vi "DiscardData.vi"(8 "error in (no err)":errorcluster caption="entrée d'erreur (pas d'erreur)", 11 "Interface In":refnum<class "Interface.lvclass"> caption="DNL_LabVIEW Object in") -> (0 "error out":errorcluster caption="sortie d'erreur", 3 "Interface Out":refnum<class "Interface.lvclass"> caption="DNL_LabVIEW Object out")   [LabVIEW 2019, in "Interface.lvclass"]
uses:
  Interface.lvclass
  Interface.lvclass/Interface.ctl
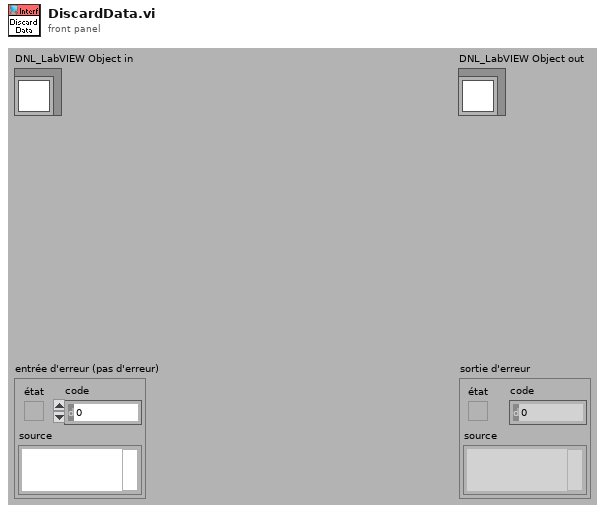
[diagram p1: front panel]
types:
  T1 = typedef "Interface.lvclass/CurveSetup.ctl" = cluster{"CurveName":string, "YParam":string, "XParam":string, "ZParam ":string, "GroupName":string, "LinWdth":u8, "PntCol":u32, "LinCol":u32, "LablFor":u8, "XScale":u32, "YScale":u32, "Interpol":u8, "DisplayName":string, "FillType":i16, "LineStyle":u8, "PntStyle":u8, "BarTyp":u8, "GraphIndex":i32, "Visible":bool, "XScaleName":string, "YScaleName":string, "XYGraph_Ref":refnum<vi>, "Data Only":bool, "DataQ Ref":refnum<queue>, "XParQ Ref":refnum<queue>, "XParamInd":i32, "ScanInd":i32, "File Path":path}
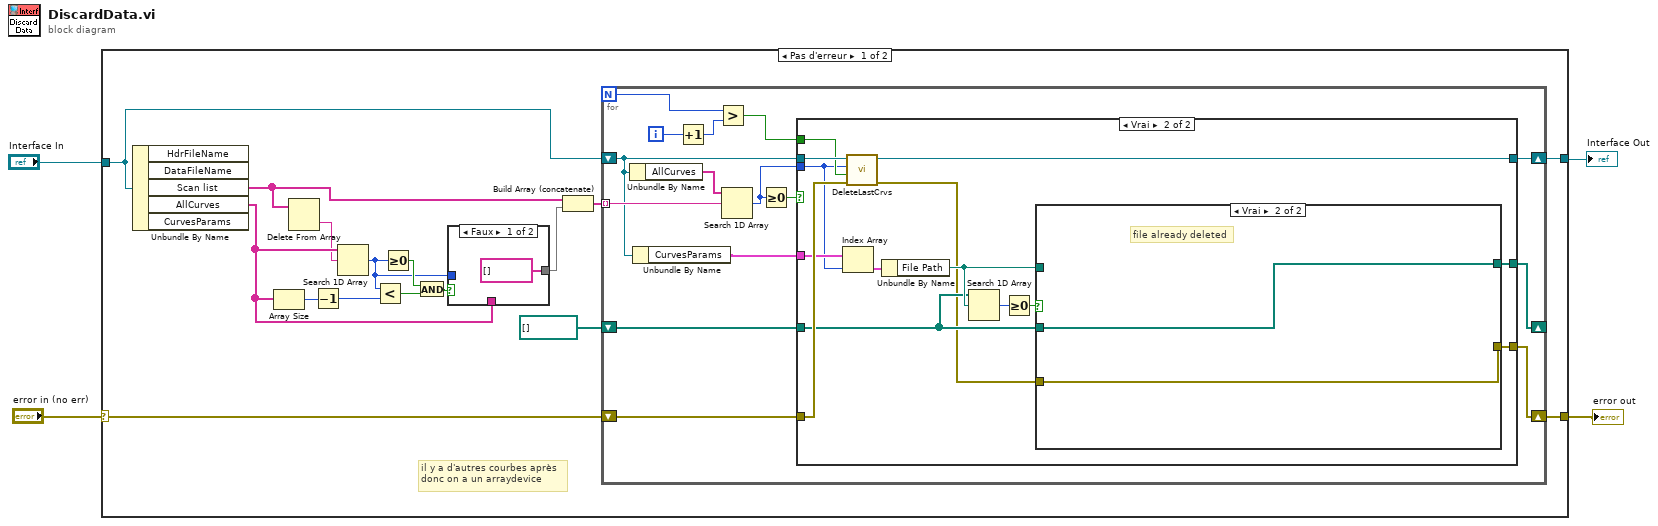
[diagram p0: block diagram]
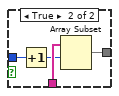
[diagram p2: hidden frame]
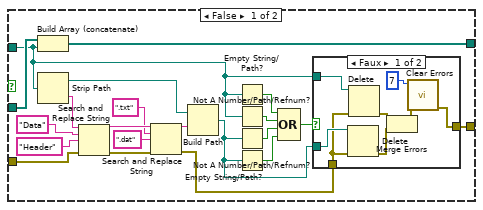
[diagram p4: hidden frame]
diagram:
  n1 = case shown="Pas d'erreur" "error in (no err)" {
    selector: "error in (no err)" -> [w18 w91]
    tunnel: [w11 w91] -> w3
    tunnel: [w19 w90] -> w1
    tunnel: "Interface In" -> [w20 w90]
    frame No Error {
      # "il y a d'autres courbes après\ndonc on a un arraydevice"
      n2 = Unbundle By Name(w20) -> ("Scan list"=w10:string[], "AllCurves"=w15:string[])  [unwired: 3 out]
      n3 = Array Size(array=w15) -> (size(s)=w17:i32)
      n4 = Delete From Array(array=w10) -> (deleted portion=w9:string)  [unwired: 2 in, 1 out]
      n5 = Decrement(x=w17) -> (x-1=w16:i32)
      n6 = Search 1D Array(1D array=w15, element=w9) -> (index of element=w5:i32)  [unwired: 1 in]
      n7 = Less?(x=w5, y=w16) -> (x < y?=w7:bool)
      n8 = Greater Or Equal To 0?(x=w5) -> (x >= 0?=w6:bool)
      n9 = And(x=w6, y=w7) -> (x .and. y?=w8:bool)
      n10 = case shown="Faux" w8 {
        tunnel: w15 -> [_ w25]
        tunnel: w5 -> [_ w24]
        tunnel: [string[] [] w22] -> w13
        frame False {
        }
        frame True {
          n11 = Increment(x=w24) -> (x+1=w23:i32)
          n12 = Array Subset(array=w25, index=w23) -> (w22:string[])  [unwired: 1 in]
        }
      }
      n13 = Build Array (concatenate)(w10, w13) -> (w14:string[])
      n14 = for {
        N -> [w34]
        shift-right: [w40] -> w19
        shift-left: w20 -> [w27]
        shift-right: [w39] -> w11
        shift-left: w18 -> [w38]
        tunnel: w14 -> [w35] mode=indexing
        shift-right: [w29] -> _
        shift-left: path[] [] -> [w28]
        i -> [w32]
        n15 = Unbundle By Name(w27) -> ("AllCurves"=w36:string[])
        n16 = Unbundle By Name(w27) -> ("CurvesParams"=w26:T1[])
        n17 = Increment(x=w32) -> (x+1=w31:i32)
        n18 = Greater?(x=w34, y=w31) -> (0:w33:bool)
        n19 = Search 1D Array(1D array=w36, element=w35) -> (index of element=w30:i32)  [unwired: 1 in]
        n20 = Greater Or Equal To 0?(x=w30) -> (x >= 0?=w37:bool)
        n21 = case shown="Vrai" w37 {
          tunnel: w27 -> [w43 w56]
          tunnel: [w43 w55] -> w40
          tunnel: w30 -> [_ w51]
          tunnel: [w42 w44] -> w39
          tunnel: w38 -> [w42 w57]
          tunnel: w33 -> [_ w54]
          tunnel: w26 -> [_ w52]
          tunnel: [w41 w50] -> w29
          tunnel: w28 -> [w41 w46]
          frame False {
            # "already deleted"
          }
          frame True {
            n22 = Index Array(array=w52, index=w51) -> (element=w53:T1)
            n23 = call "DeleteLastCrvs.vi"("error in (no error)"=w57, "defer update"=w54, "CurveNumber"=w51, "Interface en entrée"=w56) -> ("error out"=w45:errorcluster, "Interface en sortie"=w55:refnum<class "Interface.lvclass">)  [unwired: 6 in]
            n24 = Unbundle By Name(w53) -> ("File Path"=w47:path)
            n25 = Search 1D Array(1D array=w46, element=w47) -> (index of element=w49:i32)  [unwired: 1 in]
            n26 = Greater Or Equal To 0?(x=w49) -> (x >= 0?=w48:bool)
            n27 = case shown="Vrai" w48 {
              tunnel: [w78 w89] -> w50
              tunnel: w47 -> [w61 _]
              tunnel: w46 -> [w77 w89]
              tunnel: w45 -> [w67 w88]
              tunnel: [w58 w88] -> w44
              frame False {
                n28 = Build Array (concatenate)(w77, w61) -> (w78:path[])
                n29 = Strip Path(path=w61) -> (stripped path=w76:path, name=w72:string)
                n30 = Search and Replace String(input string=w72, search string="Data" ("sous-chaîne (\"\")"), replace string="Header" ("chaîne de remplacement (\"\")"), error in=w67) -> (result string=w74:string, error out=w73:errorcluster)  [unwired: 4 in, 2 out]
                n31 = Search and Replace String(input string=w74, search string=".txt" ("chaîne recherchée"), replace string=".dat" ("chaîne de remplacement (\"\")"), error in=w73) -> (result string=w75:string, error out=w59:errorcluster)  [unwired: 4 in, 2 out]
                n32 = Build Path(base path=w76, name or relative path=w75) -> (appended path=w60:path)
                n33 = Empty String/Path?(string/path=w61) -> (empty?=w63:bool)
                n34 = Not A Number/Path/Refnum?(number/path/refnum=w61) -> (NaN/Path/Refnum?=w65:bool)
                n35 = Not A Number/Path/Refnum?(number/path/refnum=w60) -> (NaN/Path/Refnum?=w66:bool)
                n36 = Empty String/Path?(string/path=w60) -> (empty?=w62:bool)
                n37 = Compound Arithmetic op=OR(w63, w65, w66, w62) -> (w64:bool)
                n38 = case shown="Faux" w64 {
                  tunnel: w61 -> [w86 _]
                  tunnel: w60 -> [w85 _]
                  tunnel: [w81 w87] -> w58
                  tunnel: w59 -> [w82 w87]
                  frame False {
                    n39 = Delete(path (use dialog)=w85, error in=w82) -> (error out=w83:errorcluster)  [unwired: 3 in, 2 out]
                    n40 = Delete(path (use dialog)=w86, error in=w82) -> (error out=w84:errorcluster)  [unwired: 3 in, 2 out]
                    n41 = Merge Errors(w84, w83) -> (w80:errorcluster)
                    n42 = call <vilib>:"Clear Errors.vi"("error in (no error)"=w80, "specific error code to clear (0: all)"=7) -> ("error out"=w81:errorcluster)  [unwired: 4 in, 1 out]
                  }
                  frame True {
                  }
                }
              }
              frame True {
                # "file already deleted"
              }
            }
          }
        }
      }
    }
    frame Error {
    }
  }
  "error out" <- w3
  "Interface Out" <- w1
